vi "Get Session Info - 1Sess .vi"(8 "error in":errorcluster, 11 "session reservation in":refnum<class "Session Reservation.lvclass">) -> (0 "error out":errorcluster, 2 "session info":T1, 3 "session reservation out":refnum<class "Session Reservation.lvclass">)   [LabVIEW 2020, in "MeasurementLink Session Management V1.lvlib" / "Session Reservation.lvclass"]
doc: "Gets the session information for the session reservation. Returns an error if the session reservation has more than one session."
uses:
  Session Reservation.lvclass
  Generated/Measurement Plugin Session Management Client/RPC Messages/ni_measurementlink_sessionmanagement_v1_SessionInformation.ctl
  Generated/Measurement Plugin Session Management Client/RPC Messages/nidevice_grpc_Session.ctl
  Generated/Measurement Plugin Session Management Client/RPC Messages/ni_measurementlink_sessionmanagement_v1_ChannelMapping.ctl
  Session Reservation.lvclass/Session Reservation.ctl
  Merge Invalid DVR Error.vi
  Is DVR Valid.vi
  MeasurementLink Measurement Server/Helpers/Error Strings Global Internal.vi
  Generated/Measurement Plugin Session Management Client/MeasurementLink Session Management Client.lvlib
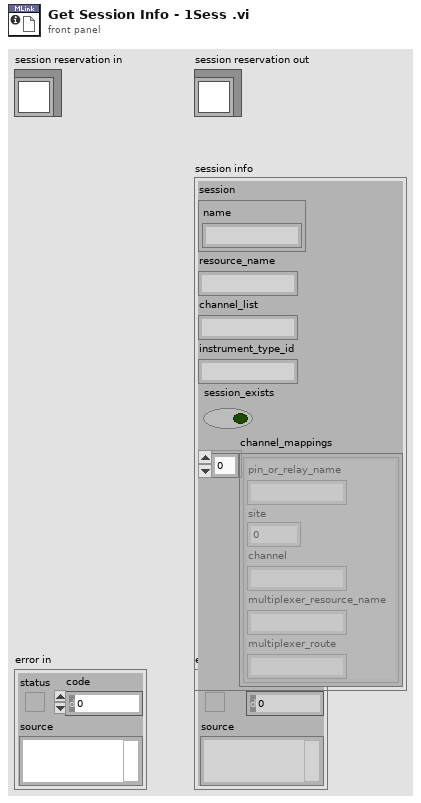
[diagram p1: front panel]
types:
  T1 = typedef "MeasurementLink Session Management Client.lvlib/ni_measurementlink_sessionmanagement_v1_SessionInformation.ctl" = cluster{"session":T2, "resource_name":string, "channel_list":string, "instrument_type_id":string, "session_exists":bool, "channel_mappings":T3[]}
  T2 = typedef "MeasurementLink Session Management Client.lvlib/nidevice_grpc_Session.ctl" = cluster{"name":string}
  T3 = typedef "MeasurementLink Session Management Client.lvlib/ni_measurementlink_sessionmanagement_v1_ChannelMapping.ctl" = cluster{"pin_or_relay_name":string, "site":i32, "channel":string, "multiplexer_resource_name":string, "multiplexer_route":string}
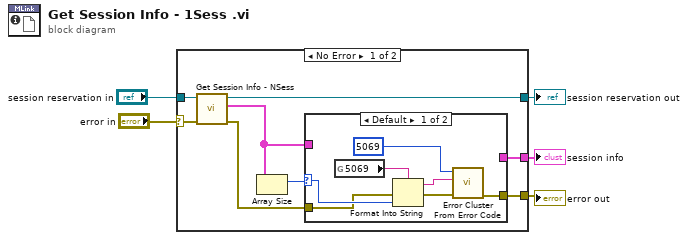
[diagram p0: block diagram]
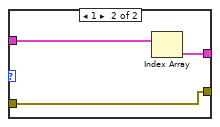
[diagram p2: hidden frame]
diagram:
  n1 = case shown="No Error" "error in" {
    selector: "error in" -> [w6 w25]
    tunnel: [w12 w25] -> w5
    tunnel: [w11 _] -> w4
    tunnel: "session reservation in" -> [w10 w24]
    tunnel: [w9 w24] -> w2
    frame No Error {
      n2 = call "Get Session Info - NSess .vi"("error in"=w6, "session reservation in"=w10) -> ("error out"=w7:errorcluster, "sessions info"=w8:T1[], "session reservation out"=w9:refnum<class "Session Reservation.lvclass">)  [unwired: 7 in]
      n3 = Array Size(array=w8) -> (size(s)=w13:i32)
      n4 = case shown="Default" w13 {
        selector: w13 -> [w15 _]
        tunnel: w8 -> [_ w23]
        tunnel: [_ w22] -> w11
        tunnel: [w20 w21] -> w12
        tunnel: w7 -> [w14 w21]
        frame Default {
          n5 = global read "Error Strings Global Internal.vi" "5069"() -> (w16:string)
          n6 = Format Into String(format string=w16, error in=w14, w15) -> (resulting string=w17:string, error out=w18:errorcluster)  [unwired: 1 in]
          n7 = call <vilib>:"Error Cluster From Error Code.vi"("error in (no error)"=w18, "error message (\"\")"=w17, "error code (0)"=5069) -> ("error out"=w20:errorcluster)  [unwired: 6 in]
        }
        frame 1 {
          n8 = Index Array(array=w23) -> (element=w22:T1)  [unwired: 1 in]
        }
      }
    }
    frame Error {
    }
  }
  "error out" <- w5
  "session reservation out" <- w2
  "session info" <- w4
